vi "Attached Camera Info AE.vi"(7 "update":bool, 9 "InterfaceName":string, 11 "Camera Information Array":T1(array[cluster]) {"BusType" format="%x"; "SerialNumberLow" format="%.0x"; "SerialNumberHigh" format="%.0x"}) -> (2 "Serial Number":string)   [LabVIEW 2025]
panel:
  out "Serial Number 2":string
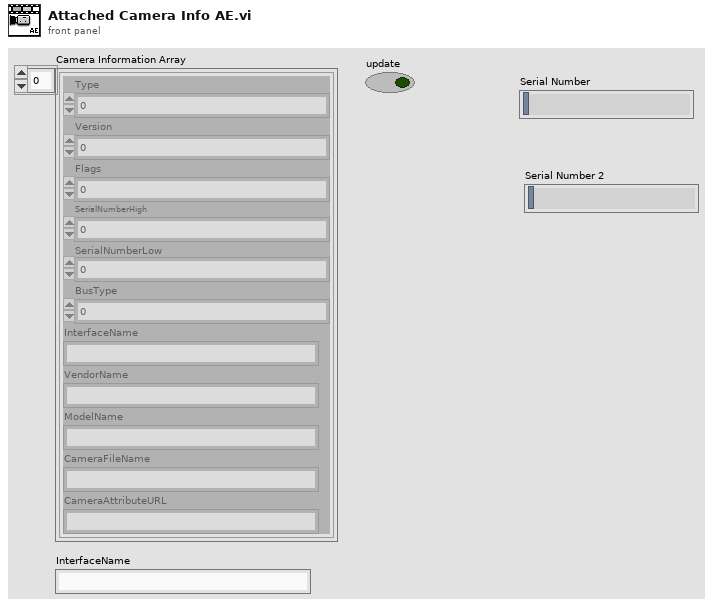
[diagram p1: front panel]
types:
  T1 = cluster{"Type":u32, "Version":u32, "Flags":u32, "SerialNumberHigh":u32, "SerialNumberLow":u32, "BusType":u32, "InterfaceName":string, "VendorName":string, "ModelName":string, "CameraFileName":string, "CameraAttributeURL":string}[]
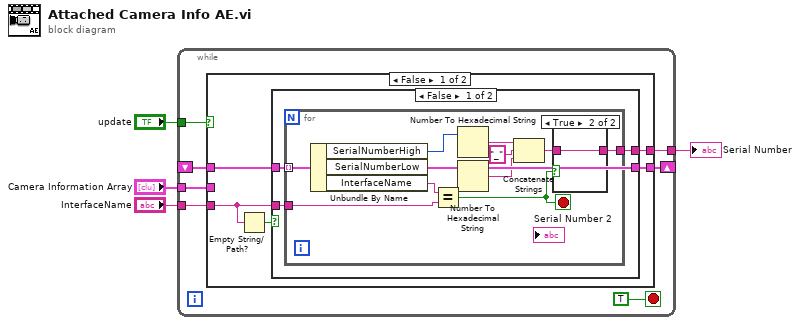
[diagram p0: block diagram]
diagram:
  n1 = while {
    tunnel: "InterfaceName" -> [w10]
    tunnel: [w9] -> w3
    tunnel: "update" -> [w8]
    shift-right: [w7] -> _
    shift-left: _ -> [w5]
    tunnel: "Camera Information Array" -> [w6]
    stop <- TRUE stop-if-true
    n2 = case shown="False" w8 {
      tunnel: w10 -> [w15 _]
      tunnel: [w14 _] -> w9
      tunnel: [w12 w33] -> w7
      tunnel: w6 -> [_ w33]
      tunnel: w5 -> [w13 _]
      frame False {
        n3 = Empty String/Path?(string/path=w15) -> (empty?=w16:bool)
        n4 = case shown="False" w16 {
          tunnel: w13 -> [w17 w32]
          tunnel: w15 -> [w19 _]
          tunnel: [w18 _] -> w14
          tunnel: [w17 w32] -> w12
          frame False {
            n5 = for {
              tunnel: w17 -> [w30] mode=indexing
              tunnel: w19 -> [w28]
              tunnel: [w22] -> w18
              stop <- w21 stop-if-true
              n6 = Unbundle By Name(w30) -> ("SerialNumberHigh"=w27:u32, "SerialNumberLow"=w26:u32, "InterfaceName"=w29:string)
              n7 = Equal?(x=w29, y=w28) -> (x = y?=w21:bool)
              n8 = Number To Hexadecimal String(2:w27) -> (0:w25:string)  [unwired: 1 in]
              n9 = Number To Hexadecimal String(2:w26) -> (0:w24:string)  [unwired: 1 in]
              n10 = Concatenate Strings(w25, "_" ("string"), w24) -> (w23:string)
              n11 = case shown="True" w21 {
                tunnel: w23 -> [_ w31]
                tunnel: [_ w31] -> w22
                frame False {
                }
                frame True {
                }
              }
            }
          }
          frame True {
          }
        }
      }
      frame True {
      }
    }
  }
  "Serial Number" <- w3
